vi "Untitled 1 (SubVI).vi"(8 "error in (no error)":errorcluster, 10 "Python File":path, 11 "session in":refnum<k35>) -> (0 "error out":errorcluster, 1 "Array":i32[](array[numeric]), 2 "Map":map{string, dbl}(c390), 3 "session out":refnum<k35>)   [LabVIEW 2024]
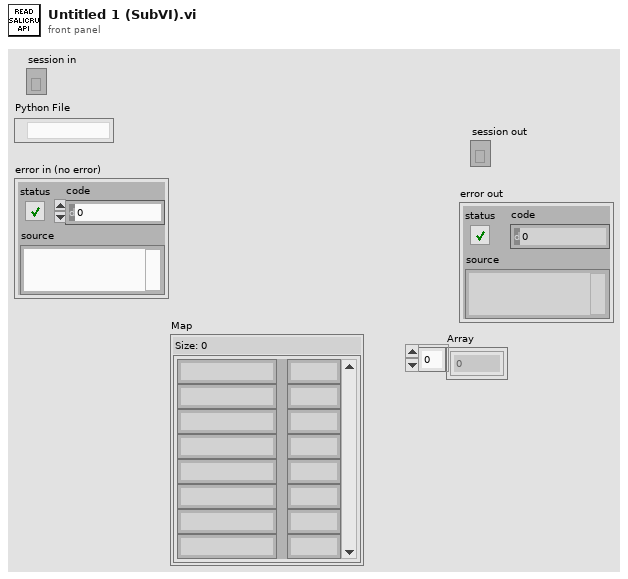
[diagram p1: front panel]
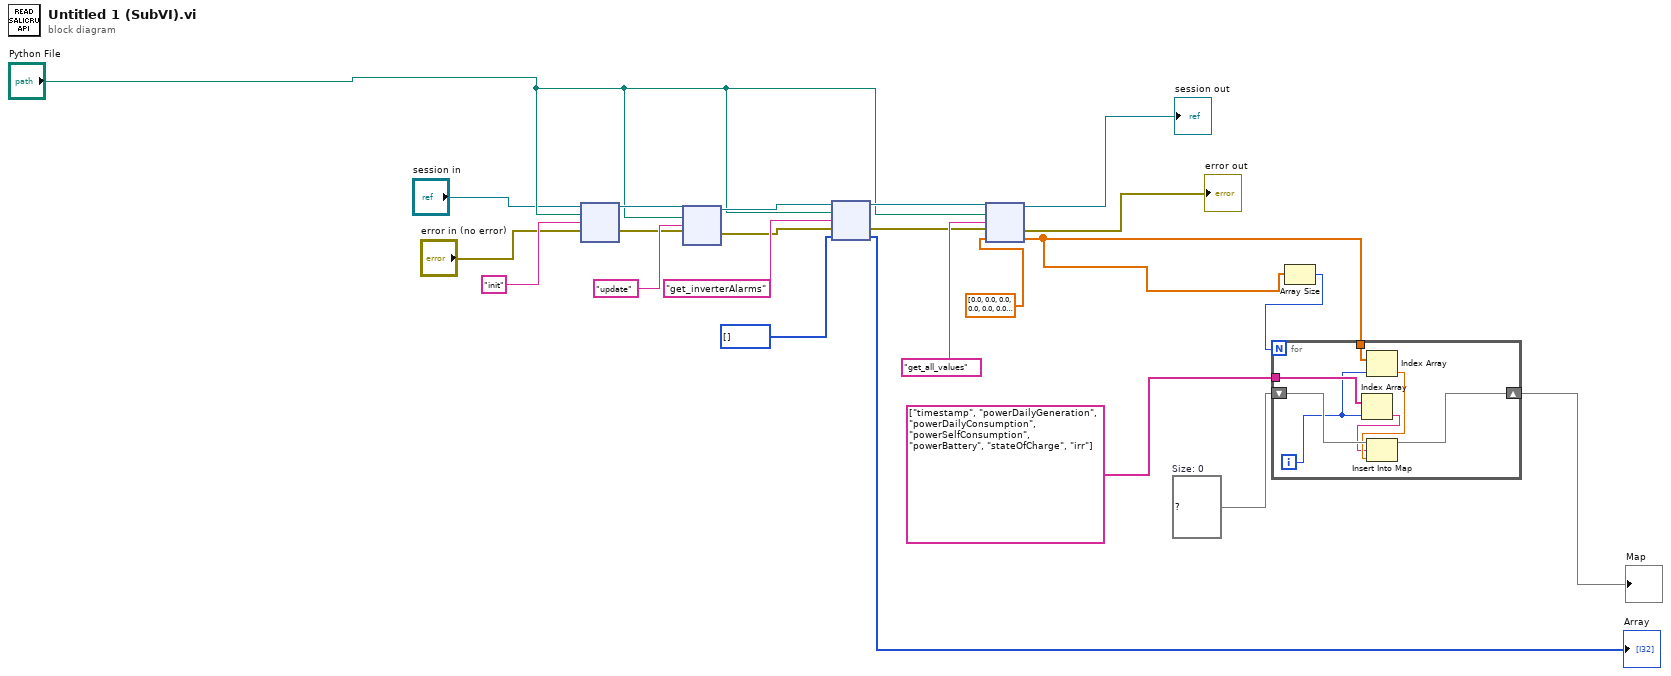
[diagram p0: block diagram]
diagram:
  w20 = map{string, dbl} {}  # Size: 0
  n1 = node("session in", "Python File", "init" ("function name"), "error in (no error)") -> (w7:refnum<k35>, w8:errorcluster)  [unwired: 2 in, 2 out]
  n2 = node(w7, "Python File", "update" ("function name"), w8) -> (w10:refnum<k35>, w11:errorcluster)  [unwired: 2 in, 2 out]
  n3 = node(w10, "Python File", "get_inverterAlarms" ("function name"), w11, i32[] []) -> (w13:refnum<k35>, w14:errorcluster, →"Array":i32[])  [unwired: 2 out]
  n4 = node(w13, "Python File", "get_all_values" ("function name"), w14, dbl[] [0.0, 0.0, 0.0, 0.0, 0.0, 0.0, 0.0, 0.0]) -> (→"session out":refnum<k35>, →"error out":errorcluster, w21:dbl[])  [unwired: 2 out]
  n5 = Array Size(array=w21) -> (size(s)=w19:i32)
  n6 = for {
    N: w19 -> [_]
    shift-right: [w30] -> w23
    shift-left: w20 -> [w29]
    tunnel: w21 -> [w28]
    tunnel: string[] ["timestamp", "powerDailyGeneration", "powerDailyConsumption", "powerSelfConsumption", "powerBattery", "stateOfCharge", "irr"] -> [w27]
    i -> [w26]
    n7 = Index Array(array=w27, index=w26) -> (element=w24:string)
    n8 = Index Array(array=w28, index=w26) -> (element=w25:dbl)
    n9 = Insert Into Map(map in=w29, key=w24, value=w25) -> (map out=w30:map{string, dbl})  [unwired: 2 out]
  }
  "Map" <- w23
